vi "Initialize Channel Data.vi"(8 "error in (no error)":errorcluster, 9 "FIFOs":T1, 10 "Engine Data in":T3, 11 "Device Ref in":T2 format="%.0x") -> (0 "error out":errorcluster, 2 "Engine Data out":T3, 3 "Device Ref out":T2 format="%.0x")   [LabVIEW 2017, in "Routing and Faulting Engine.lvlib"]
uses:
  Routing and Faulting Engine.lvlib
  <vilib>/NI Veristand/Custom Device API/Custom Device Item Ref.ctl
  Engine Data.ctl
  Includes/CDMessaging.lvlibp/Producer/Abstract Producer/Abstract Producer.lvclass
  Shared/Compiled.Settings.ctl
  Shared/Communication Configuration.ctl
  Shared/Routing and Faulting Configuration.ctl
  Shared/Routing Channel Configuration.ctl
  Shared/Value-Connections Map.ctl
  Shared/Connection.ctl
  Shared/Alias Mapping.ctl
  Shared/FIFO Indices.ctl
  Device Inputs.ctl
  Device Outputs.ctl
  Device FIFOs.ctl
  <vilib>/NI Veristand/Custom Device API/Custom Device Channel Type.ctl
  <vilib>/NI Veristand/Custom Device API/Custom Device API.lvlib
  Shared/Routing and Faulting Shared.lvlib
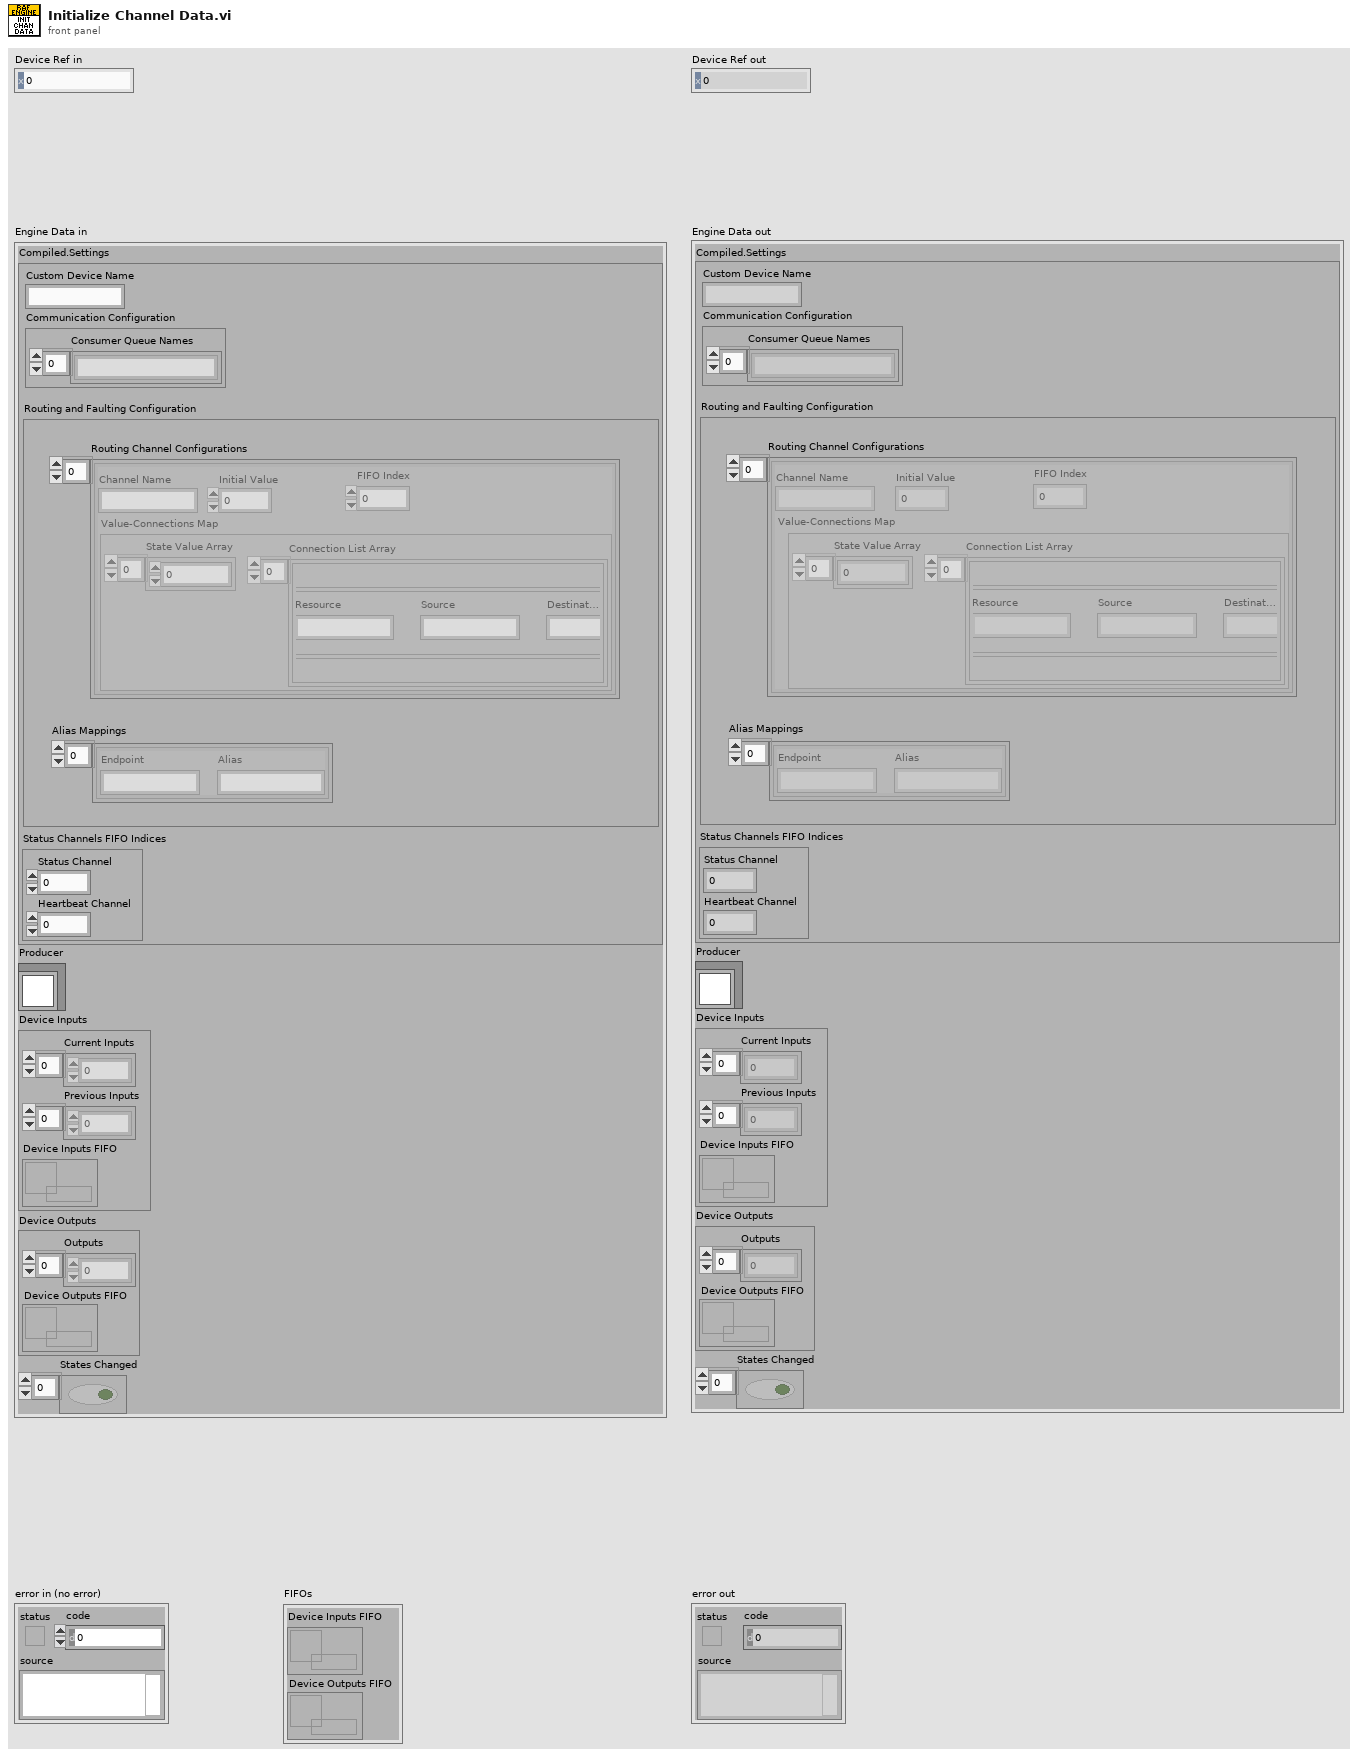
[diagram p1: front panel]
types:
  T1 = typedef "Routing and Faulting Engine.lvlib/Device FIFOs.ctl" = cluster{"Device Inputs FIFO":refnum<k33>, "Device Outputs FIFO":refnum<k33>}
  T2 = typedef "Custom Device API.lvlib/Custom Device Item Ref.ctl" = u64
  T3 = typedef "Routing and Faulting Engine.lvlib/Engine Data.ctl" = cluster{"Compiled.Settings":T4, "Producer":refnum<class "Abstract Producer.lvclass">, "Device Inputs":T12, "Device Outputs":T13, "States Changed":bool[]}
  T4 = typedef "Routing and Faulting Shared.lvlib/Compiled.Settings.ctl" = cluster{"Custom Device Name":string, "Communication Configuration":T5, "Routing and Faulting Configuration":T6, "Status Channels FIFO Indices":T11}
  T5 = typedef "Routing and Faulting Shared.lvlib/Communication Configuration.ctl" = cluster{"Consumer Queue Names":string[]}
  T6 = typedef "Routing and Faulting Shared.lvlib/Routing and Faulting Configuration.ctl" = cluster{"Routing Channel Configurations":T7[], "Alias Mappings":T10[]}
  T7 = typedef "Routing and Faulting Shared.lvlib/Routing Channel Configuration.ctl" = cluster{"Channel Name":string, "Initial Value":dbl, "FIFO Index":i32, "Value-Connections Map":T8}
  T8 = typedef "Routing and Faulting Shared.lvlib/Value-Connections Map.ctl" = cluster{"State Value Array":i32[], "Connection List Array":cluster{"Connection List":T9[]}[]}
  T9 = typedef "Routing and Faulting Shared.lvlib/Connection.ctl" = cluster{"Resource":string, "Source":string, "Destination":string}
  T10 = typedef "Routing and Faulting Shared.lvlib/Alias Mapping.ctl" = cluster{"Endpoint":string, "Alias":string}
  T11 = typedef "Routing and Faulting Shared.lvlib/FIFO Indices.ctl" = cluster{"Status Channel":i32, "Heartbeat Channel":i32}
  T12 = typedef "Routing and Faulting Engine.lvlib/Device Inputs.ctl" = cluster{"Current Inputs":dbl[], "Previous Inputs":dbl[], "Device Inputs FIFO":refnum<k33>}
  T13 = typedef "Routing and Faulting Engine.lvlib/Device Outputs.ctl" = cluster{"Outputs":dbl[], "Device Outputs FIFO":refnum<k33>}
  T14 = typedef "Custom Device API.lvlib/Custom Device Channel Type.ctl" = enum16{"Input", "Output"}
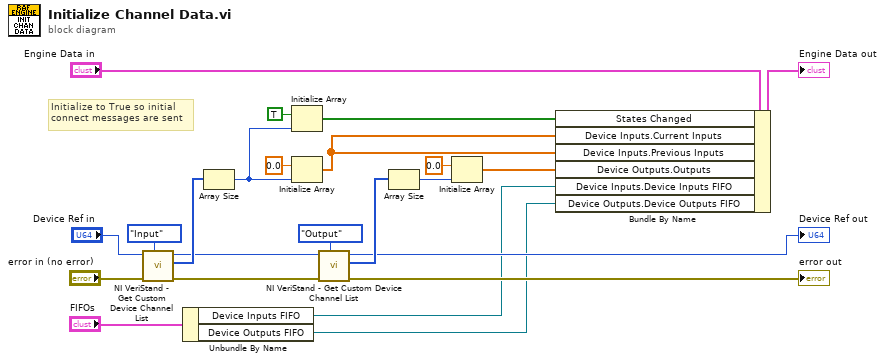
[diagram p0: block diagram]
diagram:
  # "Initialize to True so initial\nconnect messages are sent"
  n1 = call <vilib>:"NI VeriStand - Get Custom Device Channel List.vi"("Channel Type"=Custom_Device_Channel_Type."Input", "error in (no error)"="error in (no error)", "Device Ref in"="Device Ref in") -> ("error out"=w17:errorcluster, "Specified Channel Ref List"=w23:T2[], "Device Ref out"=w12:T2)  [unwired: 6 out]
  n2 = Unbundle By Name("FIFOs") -> ("Device Inputs FIFO"=w4:refnum<k33>, "Device Outputs FIFO"=w6:refnum<k33>)
  n3 = Array Size(array=w23) -> (size(s)=w2:i32)
  n4 = Initialize Array(TRUE, w2) -> (w1:bool[])
  n5 = Initialize Array(0.0 ("element"), w2) -> (w8:dbl[])
  n6 = call <vilib>:"NI VeriStand - Get Custom Device Channel List.vi"("Channel Type"=Custom_Device_Channel_Type."Output", "error in (no error)"=w17, "Device Ref in"=w12) -> ("error out"=→"error out":errorcluster, "Specified Channel Ref List"=w13:T2[], "Device Ref out"=→"Device Ref out":T2)  [unwired: 6 out]
  n7 = Array Size(array=w13) -> (size(s)=w14:i32)
  n8 = Initialize Array(0.0 ("element"), w14) -> (w5:dbl[])
  n9 = Bundle By Name(cluster="Engine Data in", "States Changed"=w1, "Device Inputs.Current Inputs"=w8, "Device Inputs.Previous Inputs"=w8, "Device Outputs.Outputs"=w5, "Device Inputs.Device Inputs FIFO"=w4, "Device Outputs.Device Outputs FIFO"=w6) -> (→"Engine Data out":T3)
